vi "String.2D to String.vi"(7 "DelimCol":string=";", 10 "DelimRow":string="|", 11 "Array":string[][](array[string])) -> (3 "String":string)   [LabVIEW 2019]
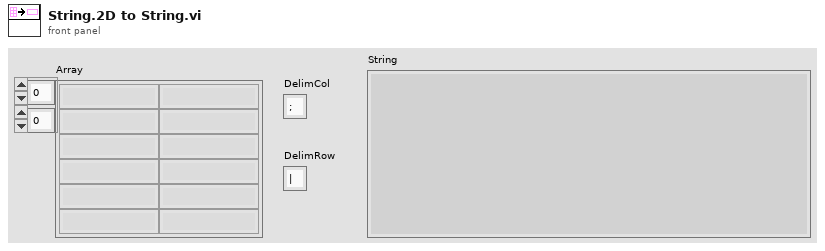
[diagram p1: front panel]
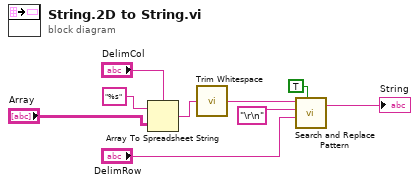
[diagram p0: block diagram]
diagram:
  n1 = Array To Spreadsheet String(delimiter (Tab)="DelimCol", array="Array", 3:"%s" ("format string")) -> (spreadsheet string=w4:string)
  n2 = call <vilib>:"Trim Whitespace.vi"("string"=w4) -> ("trimmed string"=w3:string)  [unwired: 1 in]
  n3 = call <vilib>:"Search and Replace Pattern.vi"("string"=w3, "regular expression (\"\")"="\r\n" ("regular expression (\"\")"), "replace string (\"\")"="DelimRow", "replace all? (F)"=TRUE) -> ("result string"=→"String":string)  [unwired: 1 in, 1 out]
